vi "GetFrame.vi"(8 "error in (no error)":errorcluster, 11 "ZWO_ASI in":refnum<class "ZWO_ASI.lvclass">) -> (0 "error out":errorcluster, 3 "ZWO_ASI out":refnum<class "ZWO_ASI.lvclass">)   [LabVIEW 2023, in "ZWO_ASI.lvlib" / "ZWO_ASI.lvclass"]
uses:
  ZWO_ASI.lvclass
  ZWO_ASI.lvclass/ZWO_ASI.ctl
  <userlib>/ASICamera2_no_err/ASICamera2_no_err.lvlib
  CameraDAQ Messages/GrabFrame Msg/GrabFrame Msg.lvclass
  <vilib>/ActorFramework/Actor/Actor.lvclass
  <vilib>/ActorFramework/Message Enqueuer/Message Enqueuer.lvclass
  Applications/National Instruments/LabVIEW 2023 64-bit/vi.lib/ActorFramework/Actor/Actor.lvclass
  Users/alexandrosspiliotis/Documents/ZWO_ASI/ZWO_ASI/ZWO_ASI.lvclass
  Users/alexandrosspiliotis/Documents/TranslationStage/InitDeinit/InitDeinit.lvclass
  Users/alexandrosspiliotis/Documents/OrcaLV/ImagingDevice/ImagingDevice.lvclass
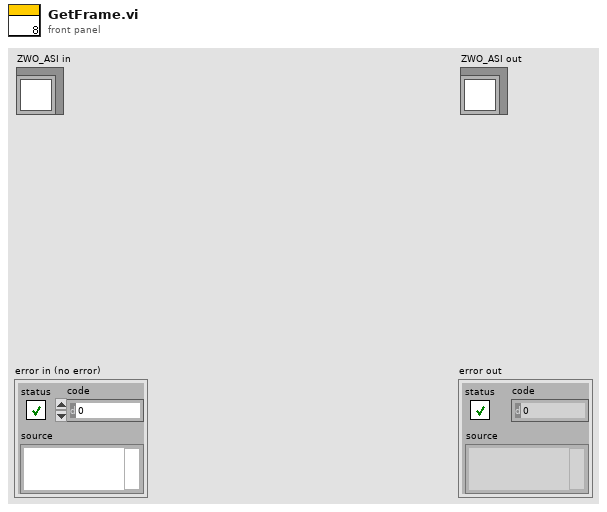
[diagram p1: front panel]
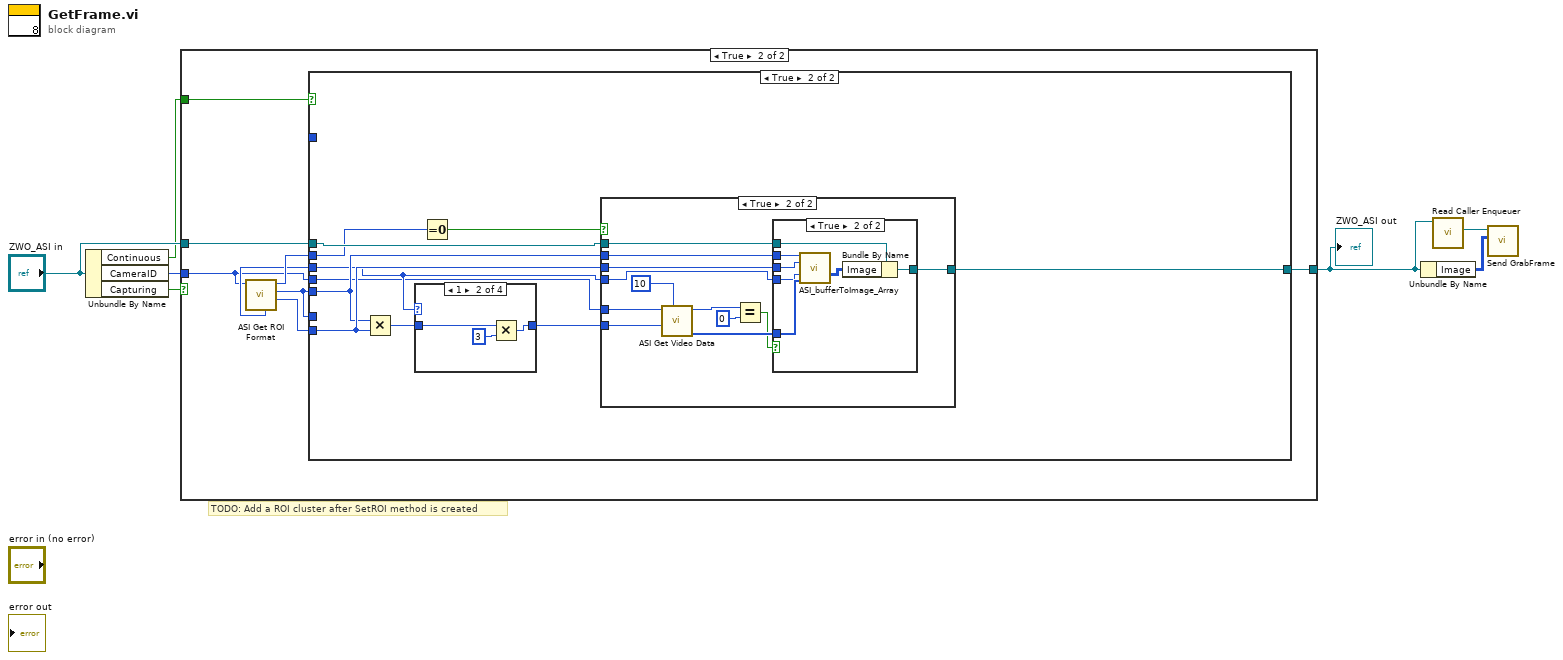
[diagram p0: block diagram]
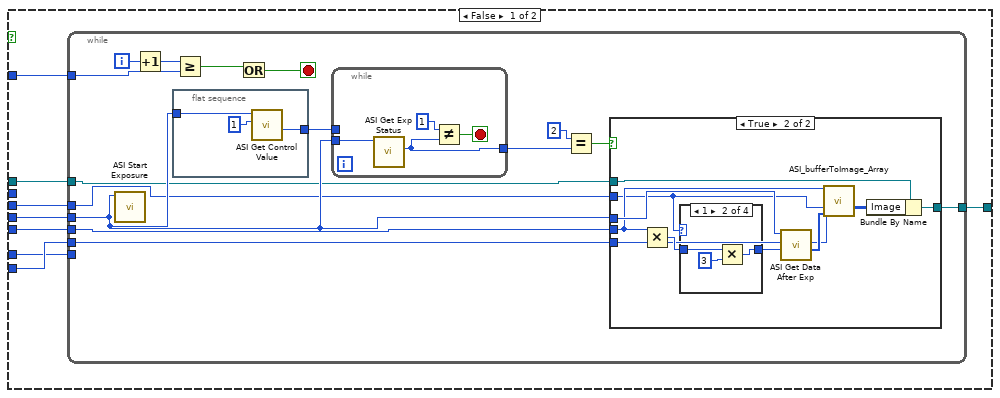
[diagram p3: hidden frame]
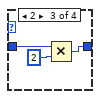
[diagram p6: hidden frame]
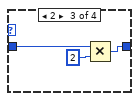
[diagram p11: hidden frame]
diagram:
  # "TODO: Add a ROI cluster after SetROI method is created"
  n1 = Unbundle By Name("ZWO_ASI in") -> ("Continuous"=w6:bool, "CameraID"=w5:i32, "Capturing"=w4:bool)
  n2 = case shown="True" w4 {
    tunnel: "ZWO_ASI in" -> [w8 w17]
    tunnel: [w8 w16] -> w2
    tunnel: w6 -> [_ w10]
    tunnel: w5 -> [_ w9]
    frame False {
    }
    frame True {
      n3 = call <userlib>:"ASI Get ROI Format.vi"("iCameraID"=w9) -> ("piHeight out"=w15:i32, "piWidth out"=w12:i32, "function return"=w14:i32, "pImg_type out"=w13:i32)  [unwired: 6 in, 1 out]
      n4 = case shown="True" w10 {
        tunnel: w17 -> [w20 w76]
        tunnel: [w19 w75] -> w16
        tunnel: w15 -> [w23 w71]
        tunnel: w12 -> [w21 w70]
        tunnel: w14 -> [_ w69]
        tunnel: w13 -> [w24 w68]
        tunnel: w9 -> [w25 w67]
        tunnel: w12 -> [w22 _]
        tunnel: [w18 _] -> w11
        frame False {
          n5 = while {
            tunnel: w25 -> [w39]
            tunnel: w21 -> [w34]
            tunnel: w24 -> [w29]
            tunnel: w23 -> [w30]
            tunnel: w22 -> [_]
            tunnel: w20 -> [w28]
            tunnel: [w27] -> w19
            tunnel: w18 -> [w26]
            i -> [w38]
            stop <- w35 stop-if-true
            n6 = call <userlib>:"ASI Start Exposure.vi"("iCameraID"=w39) -> ()  [unwired: 10 in, 1 out]
            n7 = Increment(x=w38) -> (x+1=w37:i32)
            n8 = flat-sequence {
              tunnel: w39 -> [w43]
              tunnel: [w42] -> w33
              frame #0 {
                n9 = call <userlib>:"ASI Get Control Value.vi"("ControlType"=1, "iCameraID"=w43) -> ("plValue out"=w42:i32)  [unwired: 7 in, 2 out]
              }
            }
            n10 = Greater Or Equal?(x=w37, y=w26) -> (x >= y?=w36:bool)
            n11 = Or(x=w36) -> (x .or. y?=w35:bool)  [unwired: 1 in]
            n12 = while {
              tunnel: w39 -> [w47]
              tunnel: [w44] -> w32
              tunnel: w33 -> [_]
              stop <- w45 stop-if-true
              n13 = call <userlib>:"ASI Get Exp Status.vi"("iCameraID"=w47) -> ("pExpStatus out"=w44:u32)  [unwired: 9 in, 1 out]
              n14 = Not Equal?(x=u32 1, y=w44) -> (x != y?=w45:bool)
            }
            n15 = Equal?(x=u32 2, y=w32) -> (x = y?=w40:bool)
            n16 = case shown="True" w40 {
              tunnel: w39 -> [_ w58]
              tunnel: w34 -> [_ w53]
              tunnel: w30 -> [_ w54]
              tunnel: w29 -> [_ w52]
              tunnel: w28 -> [w48 w50]
              tunnel: [w48 w51] -> w27
              frame False {
              }
              frame True {
                n17 = Multiply(x=w53, y=w54) -> (x*y=w56:i32)
                n18 = case shown="1" w52 {
                  tunnel: w56 -> [w59 w62 w65 w66]
                  tunnel: [w59 w60 w63 w66] -> w57
                  frame 0, Default {
                  }
                  frame 1 {
                    n19 = Multiply(x=w62, y=3) -> (x*y=w60:i32)
                  }
                  frame 2 {
                    n20 = Multiply(x=w65, y=2) -> (x*y=w63:i32)
                  }
                  frame 3 {
                  }
                }
                n21 = call <userlib>:"ASI Get Data After Exp.vi"("lBuffSize"=w57, "iCameraID"=w58) -> ("pBuffer out"=w55:u8[])  [unwired: 8 in, 1 out]
                n22 = call "ASI_bufferToImage_Array.vi"("iWidth"=w53, "iHeight"=w54, "imageType"=w52, "pBuffer in"=w55) -> ("output array"=w49:u32[][])  [unwired: 11 in]
                n23 = Bundle By Name(cluster=w50, "Image"=w49) -> (w51:refnum<class "ZWO_ASI.lvclass">)
              }
            }
          }
        }
        frame True {
          n24 = Multiply(x=w70, y=w71) -> (x*y=w73:i32)
          n25 = case shown="1" w68 {
            tunnel: w73 -> [w98 w101 w104 w105]
            tunnel: [w98 w99 w102 w105] -> w74
            frame 0, Default {
            }
            frame 1 {
              n26 = Multiply(x=w101, y=3) -> (x*y=w99:i32)
            }
            frame 2 {
              n27 = Multiply(x=w104, y=2) -> (x*y=w102:i32)
            }
            frame 3 {
            }
          }
          n28 = Equal To 0?(x=w69) -> (x = 0?=w72:bool)
          n29 = case shown="True" w72 {
            tunnel: w67 -> [_ w89]
            tunnel: w76 -> [w77 w88]
            tunnel: [w77 w87] -> w75
            tunnel: w68 -> [_ w86]
            tunnel: w71 -> [_ w85]
            tunnel: w70 -> [_ w84]
            tunnel: w74 -> [_ w83]
            frame False {
            }
            frame True {
              n30 = call <userlib>:"ASI Get Video Data.vi"("iWaitms"=10, "lBuffSize"=w83, "iCameraID"=w89) -> ("pBuffer out"=w81:u8[], "function return"=w80:i32)  [unwired: 7 in]
              n31 = Equal?(x=w80, y=0) -> (x = y?=w78:bool)
              n32 = case shown="True" w78 {
                tunnel: w84 -> [_ w97]
                tunnel: w85 -> [_ w96]
                tunnel: w81 -> [_ w95]
                tunnel: w86 -> [_ w94]
                tunnel: w88 -> [w90 w93]
                tunnel: [w90 w91] -> w87
                frame False {
                }
                frame True {
                  n33 = call "ASI_bufferToImage_Array.vi"("iWidth"=w97, "iHeight"=w96, "imageType"=w94, "pBuffer in"=w95) -> ("output array"=w92:u32[][])  [unwired: 11 in]
                  n34 = Bundle By Name(cluster=w93, "Image"=w92) -> (w91:refnum<class "ZWO_ASI.lvclass">)
                }
              }
            }
          }
        }
      }
    }
  }
  "ZWO_ASI out" <- w2
  n35 = Unbundle By Name(w2) -> ("Image"=w1:u16[][])
  n36 = call <vilib>:"Read Caller Enqueuer.vi"("Actor"=w2) -> ("Caller Enqueuer"=w3:refnum<class "Message Enqueuer.lvclass">)  [unwired: 10 in]
  n37 = call "Send GrabFrame.vi"("Image"=w1, "Message Enqueuer"=w3) -> ()  [unwired: 8 in, 2 out]
